vi "SDG60ConfModulationDSBAM.vi"(5 "Frequency (1.0 Hz)":dbl=1.0 format="%#_16g", 6 "Mod wave shape (0:Sine)":u16(ring) items=["Sine", "Square", "Triangle", "Up Ramp", "Down Ramp", "Noise", "Arb"], 7 "error in (no error)":errorcluster, 8 "Internal/External (0: INT)":u16(ring) items=["Internal", "External", "Ch1", "Ch2"], 9 "Channel (1:Channel 1)":i32(ring)=1 items=["Channel 1"=1, "Channel 2"=2], 10 "VISA resource name":refnum<visa-resource-name>="USB0::0xF4EC::0x1101::SDG6XEBC5R0119::INSTR") -> (0 "error out":errorcluster, 3 "VISA resource name out":refnum<visa-resource-name>)   [LabVIEW 2018]
doc: "Selects the waveform shape, frequency, amplitude, offset, and phase for standard waveforms (including Sine, Square, Ramp, Pulse, DC and Arb).\n\nNotes: \nTo configure other parameters for pulse waveforms please run the Configure Pulse VI. \nTo configure noise waveform please run the Configure Noise VI.\nTo configure other parameters for arbitrary waveforms please run the Create Arbitrary Waveform. \nTo configure PRBS waveform please run the Configure PRBS Waveform VI."
panel:
  in  "State(T:On)":bool=TRUE
  # "DSBAM-Double-sideband amplitude modulation"
  # "Can set WFM then use this vi. No need to use CARR commands\nModulation can't be done on noise, DC (Not testing IQ as has trials)\nSet & config modulaton after setting up carrier WFM!"
  # "Modulation will be turned on, as needed to be on to change\nsettings. Done through SDG60ModulationOnOff vi"
  # "Will suppress carrier frequency spectral component, leaving only sidebands"
  # "With external, +/-5.5V is needed for full sweep modulation. For Ch1 and Ch2 the modulating channel needs to have ouptput in ON state, can only be activated via virtual keys - unreliable don't use\nstate for modulation to work"
  # "ARB can only be chosen from front panel. Noise produces strange results, would need testing"
  # "Range: 0.001Hz-1 MHz\n11 digit precision"
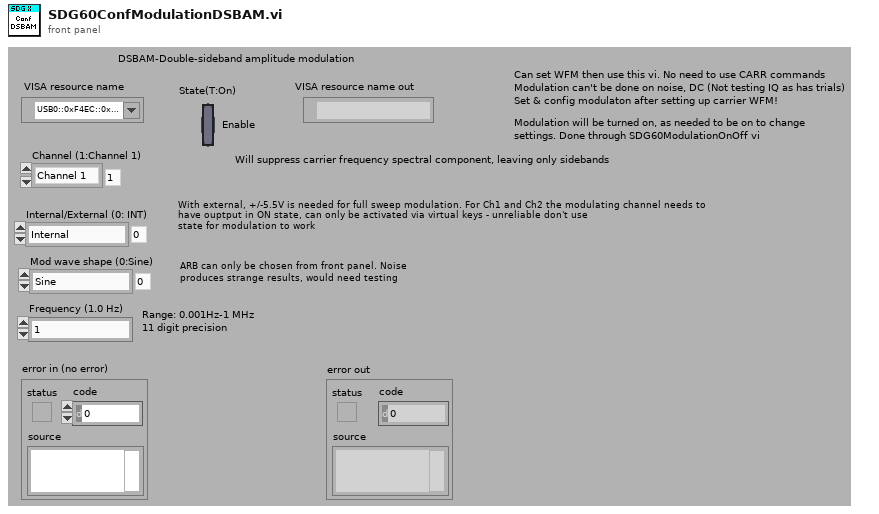
[diagram p1: front panel]
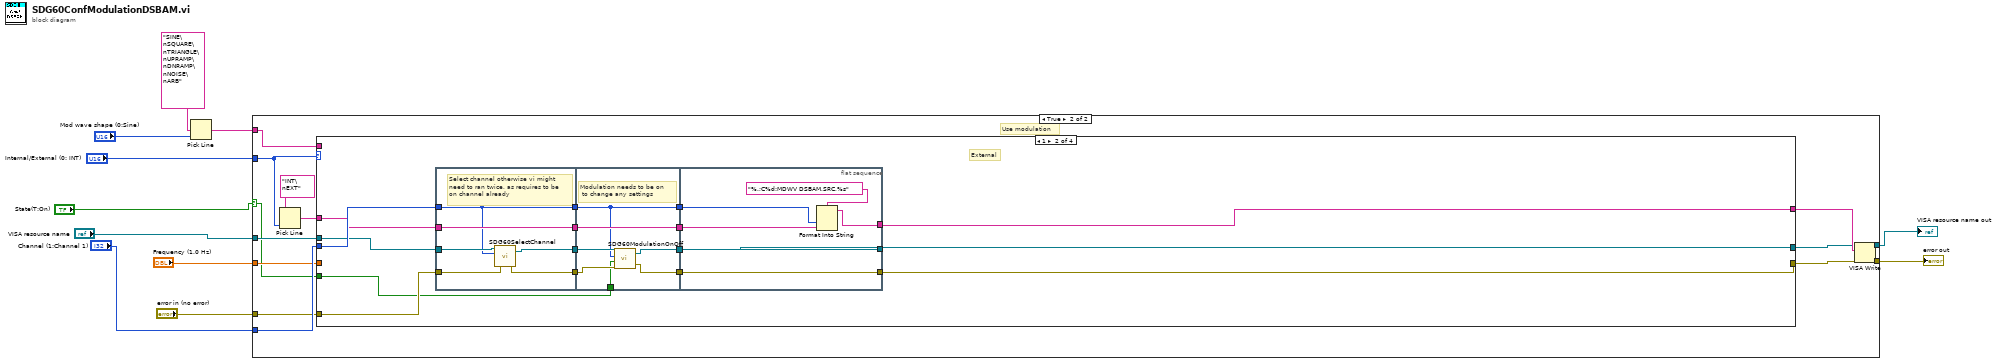
[diagram p0: block diagram]
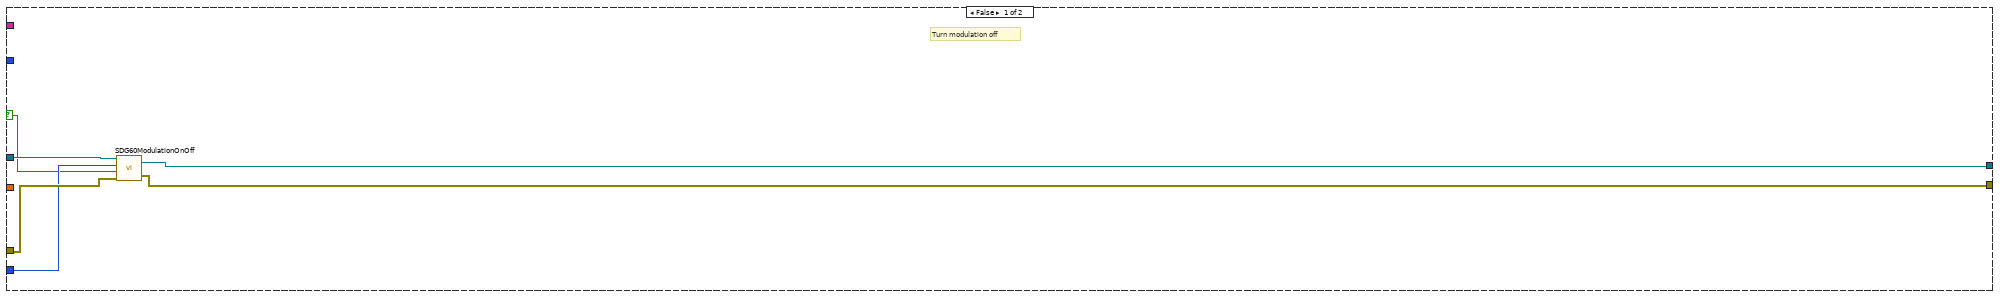
[diagram p2: hidden frame]
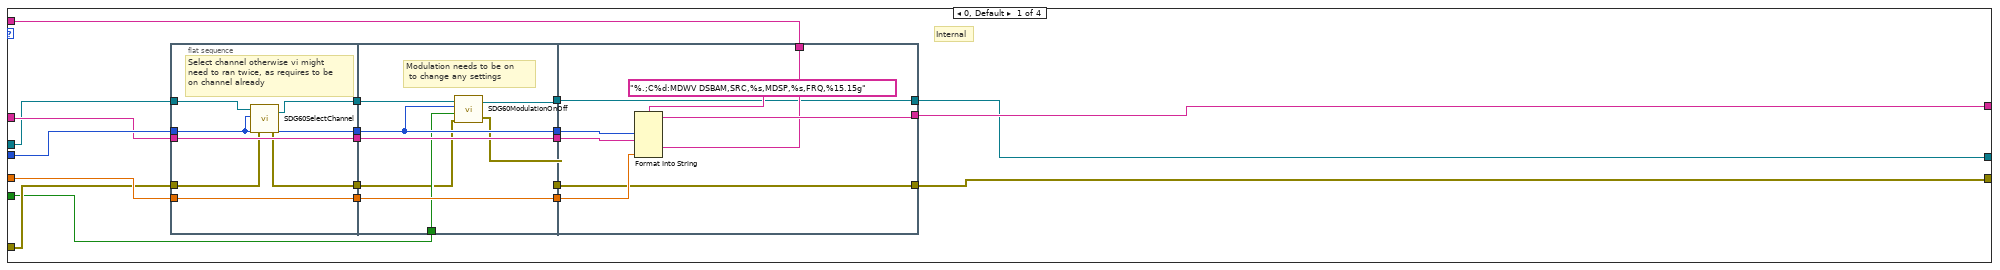
[diagram p3: hidden frame]
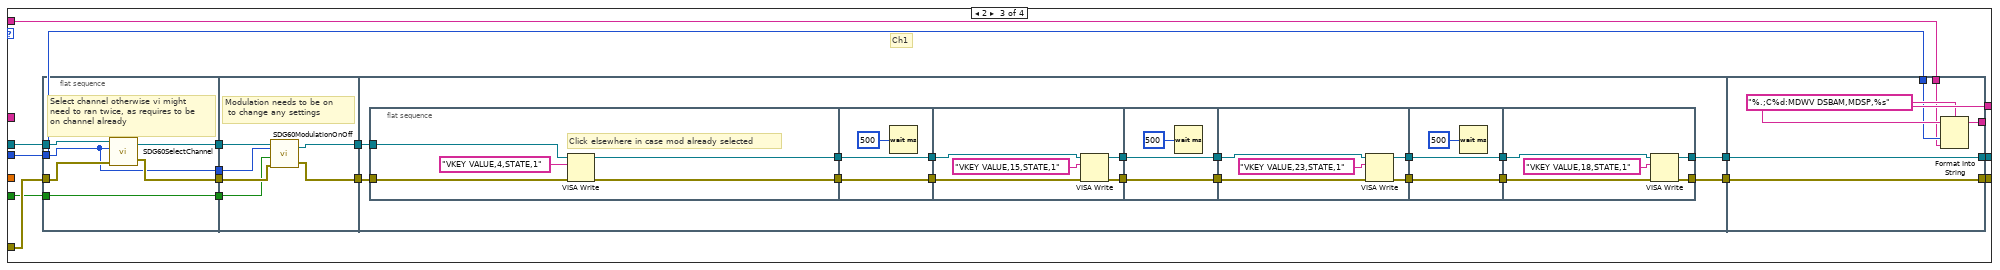
[diagram p4: hidden frame]
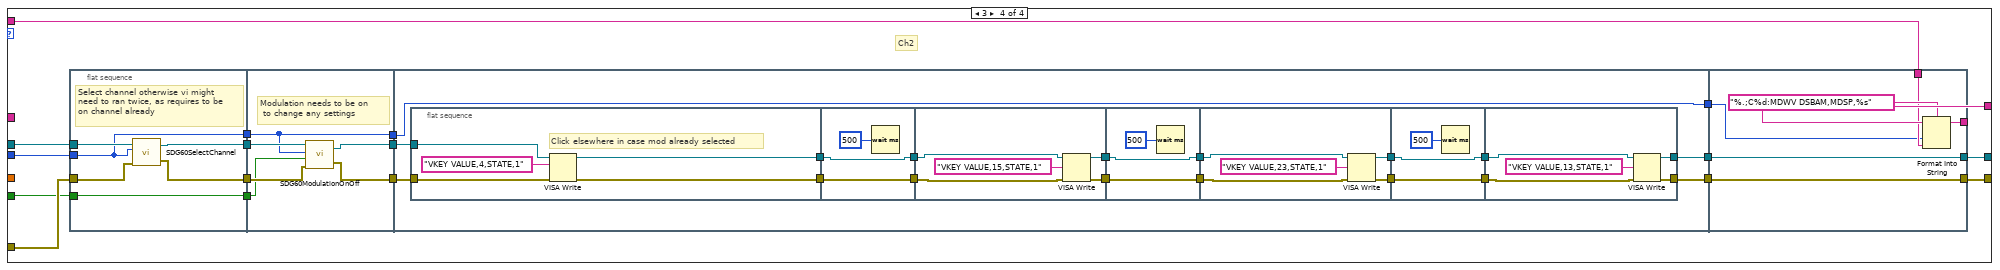
[diagram p5: hidden frame]
diagram:
  n1 = Pick Line(multi-line string="SINE\nSQUARE\nTRIANGLE\nUPRAMP\nDNRAMP\nNOISE\nARB", line index="Mod wave shape (0:Sine)") -> (output string=w6:string)  [unwired: 1 in]
  n2 = case shown="True" "State(T:On)" {
    selector: "State(T:On)" -> [w12 w18]
    tunnel: [w15 w30] -> w11
    tunnel: [w14 w29] -> w10
    tunnel: "Channel (1:Channel 1)" -> [w13 w28]
    tunnel: w6 -> [_ w27]
    tunnel: "Frequency (1.0 Hz)" -> [_ w26]
    tunnel: "VISA resource name" -> [w17 w25]
    tunnel: "error in (no error)" -> [w16 w24]
    tunnel: "Internal/External (0: INT)" -> [_ w21]
    frame False {
      # "Turn modulation off"
      n3 = call "SDG60ModulationOnOff.vi"("error in (no error)"=w16, "Enable Output (T: Enable)"=w12, "Channel (1: Channel1)"=w13, "VISA resource name"=w17) -> ("error out"=w14:errorcluster, "VISA resource name out"=w15:refnum<visa-resource-name>)
    }
    frame True {
      # "Use modulation"
      n4 = Pick Line(multi-line string="INT\nEXT", line index=w21) -> (output string=w22:string)  [unwired: 1 in]
      n5 = case shown="1" w21 {
        tunnel: [w51 w90 w121 w202] -> w31
        tunnel: w28 -> [w50 w89 w117 w198]
        tunnel: w27 -> [w49 _ w118 w199]
        tunnel: w26 -> [w48 _ _ _]
        tunnel: w25 -> [w39 w86 w123 w204]
        tunnel: w24 -> [w35 w85 w122 w203]
        tunnel: [w38 w87 w120 w201] -> w20
        tunnel: [w34 w84 w119 w200] -> w19
        tunnel: w22 -> [w47 w88 _ _]
        tunnel: w18 -> [w32 w75 w110 w193]
        frame 0, Default {
          # "Internal"
          n6 = flat-sequence {
            tunnel: w47 -> [w57]
            tunnel: w48 -> [w58]
            tunnel: w50 -> [w52]
            tunnel: [w52] -> w46
            tunnel: [w58] -> w44
            tunnel: [w57] -> w42
            tunnel: w39 -> [w56]
            tunnel: w35 -> [w53]
            tunnel: [w54] -> w36
            tunnel: [w55] -> w33
            tunnel: w46 -> [w62]
            tunnel: [w62] -> w45
            tunnel: w44 -> [w66]
            tunnel: [w66] -> w43
            tunnel: w42 -> [w65]
            tunnel: [w65] -> w41
            tunnel: [w63] -> w40
            tunnel: [w59] -> w37
            tunnel: w36 -> [w60]
            tunnel: w33 -> [w64]
            tunnel: w32 -> [w61]
            tunnel: [w73] -> w51
            tunnel: w49 -> [w71]
            tunnel: w45 -> [w72]
            tunnel: w43 -> [w70]
            tunnel: w41 -> [w69]
            tunnel: [w68] -> w38
            tunnel: w40 -> [w68]
            tunnel: [w67] -> w34
            tunnel: w37 -> [w67]
            frame #0 {
              # "Select channel otherwise vi might \nneed to ran twice, as requires to be\non channel already"
              n7 = call "SDG60SelectChannel.vi"("error in (no error)"=w53, "Channel (1: Channel1)"=w52, "VISA resource name"=w56) -> ("error out"=w54:errorcluster, "VISA resource name out"=w55:refnum<visa-resource-name>)  [unwired: 1 in]
            }
            frame #1 {
              # "Modulation needs to be on\n to change any settings"
              n8 = call "SDG60ModulationOnOff.vi"("error in (no error)"=w60, "Enable Output (T: Enable)"=w61, "Channel (1: Channel1)"=w62, "VISA resource name"=w64) -> ("error out"=w59:errorcluster, "VISA resource name out"=w63:refnum<visa-resource-name>)
            }
            frame #2 {
              n9 = Format Into String(format string="%.;C%d:MDWV DSBAM,SRC,%s,MDSP,%s,FRQ,%15.15g", w72, w69, w71, w70) -> (resulting string=w73:string)  [unwired: 2 in, 1 out]
            }
          }
        }
        frame 1 {
          # "External"
          n10 = flat-sequence {
            tunnel: w85 -> [w92]
            tunnel: w86 -> [w95]
            tunnel: w88 -> [w96]
            tunnel: w89 -> [w91]
            tunnel: [w91] -> w83
            tunnel: [w96] -> w81
            tunnel: [w94] -> w79
            tunnel: [w93] -> w77
            tunnel: w83 -> [w98]
            tunnel: [w98] -> w82
            tunnel: w81 -> [w103]
            tunnel: [w103] -> w80
            tunnel: w79 -> [w102]
            tunnel: [w101] -> w78
            tunnel: w77 -> [w99]
            tunnel: [w100] -> w76
            tunnel: w75 -> [w97]
            tunnel: [w108] -> w90
            tunnel: [w105] -> w87
            tunnel: [w104] -> w84
            tunnel: w82 -> [w107]
            tunnel: w80 -> [w106]
            tunnel: w78 -> [w105]
            tunnel: w76 -> [w104]
            frame #0 {
              # "Select channel otherwise vi might \nneed to ran twice, as requires to be\non channel already"
              n11 = call "SDG60SelectChannel.vi"("error in (no error)"=w92, "Channel (1: Channel1)"=w91, "VISA resource name"=w95) -> ("error out"=w93:errorcluster, "VISA resource name out"=w94:refnum<visa-resource-name>)  [unwired: 1 in]
            }
            frame #1 {
              # "Modulation needs to be on\n to change any settings"
              n12 = call "SDG60ModulationOnOff.vi"("error in (no error)"=w99, "Enable Output (T: Enable)"=w97, "Channel (1: Channel1)"=w98, "VISA resource name"=w102) -> ("error out"=w100:errorcluster, "VISA resource name out"=w101:refnum<visa-resource-name>)
            }
            frame #2 {
              n13 = Format Into String(format string="%.;C%d:MDWV DSBAM,SRC,%s", w107, w106) -> (resulting string=w108:string)  [unwired: 2 in, 1 out]
            }
          }
        }
        frame 2 {
          # "Ch1"
          n14 = flat-sequence {
            tunnel: w123 -> [w130]
            tunnel: w122 -> [w129]
            tunnel: [w128] -> w116
            tunnel: [w131] -> w114
            tunnel: w117 -> [w127]
            tunnel: [w127] -> w112
            tunnel: w110 -> [w126]
            tunnel: [w126] -> w111
            tunnel: w116 -> [w135]
            tunnel: [w136] -> w115
            tunnel: w114 -> [w134]
            tunnel: [w137] -> w113
            tunnel: w112 -> [w133]
            tunnel: w111 -> [w132]
            tunnel: [w148] -> w125
            tunnel: [w147] -> w124
            tunnel: w115 -> [w149]
            tunnel: w113 -> [w138]
            tunnel: [w187] -> w121
            tunnel: w125 -> [w186]
            tunnel: [w186] -> w119
            tunnel: w124 -> [w185]
            tunnel: [w185] -> w120
            tunnel: w117 -> [w184]
            tunnel: w118 -> [w183]
            frame #0 {
              # "Select channel otherwise vi might \nneed to ran twice, as requires to be\non channel already"
              n15 = call "SDG60SelectChannel.vi"("error in (no error)"=w129, "Channel (1: Channel1)"=w127, "VISA resource name"=w130) -> ("error out"=w128:errorcluster, "VISA resource name out"=w131:refnum<visa-resource-name>)  [unwired: 1 in]
            }
            frame #1 {
              # "Modulation needs to be on\n to change any settings"
              n16 = call "SDG60ModulationOnOff.vi"("error in (no error)"=w135, "Enable Output (T: Enable)"=w132, "Channel (1: Channel1)"=w133, "VISA resource name"=w134) -> ("error out"=w136:errorcluster, "VISA resource name out"=w137:refnum<visa-resource-name>)
            }
            frame #2 {
              n17 = flat-sequence {
                tunnel: w138 -> [w158]
                tunnel: [w157] -> w153
                tunnel: [w155] -> w152
                tunnel: w149 -> [w154]
                tunnel: w153 -> [w161]
                tunnel: [w161] -> w151
                tunnel: [w159] -> w150
                tunnel: w152 -> [w159]
                tunnel: w151 -> [w165]
                tunnel: w150 -> [w162]
                tunnel: [w164] -> w146
                tunnel: [w163] -> w144
                tunnel: w146 -> [w169]
                tunnel: [w169] -> w145
                tunnel: w144 -> [w168]
                tunnel: [w168] -> w143
                tunnel: w145 -> [w174]
                tunnel: w143 -> [w172]
                tunnel: [w170] -> w142
                tunnel: [w171] -> w140
                tunnel: w142 -> [w177]
                tunnel: [w177] -> w141
                tunnel: w140 -> [w176]
                tunnel: [w176] -> w139
                tunnel: [w181] -> w148
                tunnel: [w182] -> w147
                tunnel: w141 -> [w179]
                tunnel: w139 -> [w180]
                frame #0 {
                  # "Click elsewhere in case mod already selected"
                  n18 = VISA Write(VISA resource name=w158, write buffer="VKEY VALUE,4,STATE,1", error in (no error)=w154) -> (VISA resource name out=w157:refnum<visa-resource-name>, error out=w155:errorcluster)  [unwired: 1 out]
                }
                frame #1 {
                  n19 = Wait (ms)(milliseconds to wait=500) -> ()  [unwired: 1 out]
                }
                frame #2 {
                  n20 = VISA Write(VISA resource name=w165, write buffer="VKEY VALUE,15,STATE,1", error in (no error)=w162) -> (VISA resource name out=w164:refnum<visa-resource-name>, error out=w163:errorcluster)  [unwired: 1 out]
                }
                frame #3 {
                  n21 = Wait (ms)(milliseconds to wait=500) -> ()  [unwired: 1 out]
                }
                frame #4 {
                  n22 = VISA Write(VISA resource name=w174, write buffer="VKEY VALUE,23,STATE,1", error in (no error)=w172) -> (VISA resource name out=w170:refnum<visa-resource-name>, error out=w171:errorcluster)  [unwired: 1 out]
                }
                frame #5 {
                  n23 = Wait (ms)(milliseconds to wait=500) -> ()  [unwired: 1 out]
                }
                frame #6 {
                  n24 = VISA Write(VISA resource name=w179, write buffer="VKEY VALUE,18,STATE,1", error in (no error)=w180) -> (VISA resource name out=w182:refnum<visa-resource-name>, error out=w181:errorcluster)  [unwired: 1 out]
                }
              }
            }
            frame #3 {
              n25 = Format Into String(format string="%.;C%d:MDWV DSBAM,MDSP,%s", w184, w183) -> (resulting string=w187:string)  [unwired: 2 in, 1 out]
            }
          }
        }
        frame 3 {
          # "Ch2"
          n26 = flat-sequence {
            tunnel: w204 -> [w212]
            tunnel: w203 -> [w209]
            tunnel: [w210] -> w197
            tunnel: [w211] -> w195
            tunnel: w198 -> [w207]
            tunnel: w193 -> [w208]
            tunnel: [w208] -> w192
            tunnel: [w207] -> w191
            tunnel: w197 -> [w215]
            tunnel: [w216] -> w196
            tunnel: w195 -> [w218]
            tunnel: [w217] -> w194
            tunnel: w192 -> [w214]
            tunnel: w191 -> [w213]
            tunnel: [w213] -> w190
            tunnel: [w230] -> w206
            tunnel: [w229] -> w205
            tunnel: w196 -> [w231]
            tunnel: w194 -> [w220]
            tunnel: w190 -> [w219]
            tunnel: [w219] -> w189
            tunnel: [w269] -> w202
            tunnel: w206 -> [w268]
            tunnel: [w268] -> w200
            tunnel: w205 -> [w267]
            tunnel: [w267] -> w201
            tunnel: w199 -> [w266]
            tunnel: w189 -> [w265]
            frame #0 {
              # "Select channel otherwise vi might \nneed to ran twice, as requires to be\non channel already"
              n27 = call "SDG60SelectChannel.vi"("error in (no error)"=w209, "Channel (1: Channel1)"=w207, "VISA resource name"=w212) -> ("error out"=w210:errorcluster, "VISA resource name out"=w211:refnum<visa-resource-name>)  [unwired: 1 in]
            }
            frame #1 {
              # "Modulation needs to be on\n to change any settings"
              n28 = call "SDG60ModulationOnOff.vi"("error in (no error)"=w215, "Enable Output (T: Enable)"=w214, "Channel (1: Channel1)"=w213, "VISA resource name"=w218) -> ("error out"=w216:errorcluster, "VISA resource name out"=w217:refnum<visa-resource-name>)
            }
            frame #2 {
              n29 = flat-sequence {
                tunnel: w220 -> [w240]
                tunnel: [w239] -> w235
                tunnel: [w237] -> w234
                tunnel: w231 -> [w236]
                tunnel: w235 -> [w243]
                tunnel: [w243] -> w233
                tunnel: [w241] -> w232
                tunnel: w234 -> [w241]
                tunnel: w233 -> [w247]
                tunnel: w232 -> [w244]
                tunnel: [w246] -> w228
                tunnel: [w245] -> w226
                tunnel: w228 -> [w251]
                tunnel: [w251] -> w227
                tunnel: w226 -> [w250]
                tunnel: [w250] -> w225
                tunnel: w227 -> [w256]
                tunnel: w225 -> [w254]
                tunnel: [w252] -> w224
                tunnel: [w253] -> w222
                tunnel: w224 -> [w259]
                tunnel: [w259] -> w223
                tunnel: w222 -> [w258]
                tunnel: [w258] -> w221
                tunnel: [w263] -> w230
                tunnel: [w264] -> w229
                tunnel: w223 -> [w261]
                tunnel: w221 -> [w262]
                frame #0 {
                  # "Click elsewhere in case mod already selected"
                  n30 = VISA Write(VISA resource name=w240, write buffer="VKEY VALUE,4,STATE,1", error in (no error)=w236) -> (VISA resource name out=w239:refnum<visa-resource-name>, error out=w237:errorcluster)  [unwired: 1 out]
                }
                frame #1 {
                  n31 = Wait (ms)(milliseconds to wait=500) -> ()  [unwired: 1 out]
                }
                frame #2 {
                  n32 = VISA Write(VISA resource name=w247, write buffer="VKEY VALUE,15,STATE,1", error in (no error)=w244) -> (VISA resource name out=w246:refnum<visa-resource-name>, error out=w245:errorcluster)  [unwired: 1 out]
                }
                frame #3 {
                  n33 = Wait (ms)(milliseconds to wait=500) -> ()  [unwired: 1 out]
                }
                frame #4 {
                  n34 = VISA Write(VISA resource name=w256, write buffer="VKEY VALUE,23,STATE,1", error in (no error)=w254) -> (VISA resource name out=w252:refnum<visa-resource-name>, error out=w253:errorcluster)  [unwired: 1 out]
                }
                frame #5 {
                  n35 = Wait (ms)(milliseconds to wait=500) -> ()  [unwired: 1 out]
                }
                frame #6 {
                  n36 = VISA Write(VISA resource name=w261, write buffer="VKEY VALUE,13,STATE,1", error in (no error)=w262) -> (VISA resource name out=w264:refnum<visa-resource-name>, error out=w263:errorcluster)  [unwired: 1 out]
                }
              }
            }
            frame #3 {
              n37 = Format Into String(format string="%.;C%d:MDWV DSBAM,MDSP,%s", w265, w266) -> (resulting string=w269:string)  [unwired: 2 in, 1 out]
            }
          }
        }
      }
      n38 = VISA Write(VISA resource name=w20, write buffer=w31, error in (no error)=w19) -> (VISA resource name out=w30:refnum<visa-resource-name>, error out=w29:errorcluster)  [unwired: 1 out]
    }
  }
  "error out" <- w10
  "VISA resource name out" <- w11
